vi "要进入系统的界面.vi"() -> ()   [LabVIEW 2015]
panel:
  in  "取消按钮":bool
  in  "声音来源":path=path "E:/桌面/Desktop/wav/儿童歌曲 - 葫芦娃 (儿童版).wav" caption="路径"
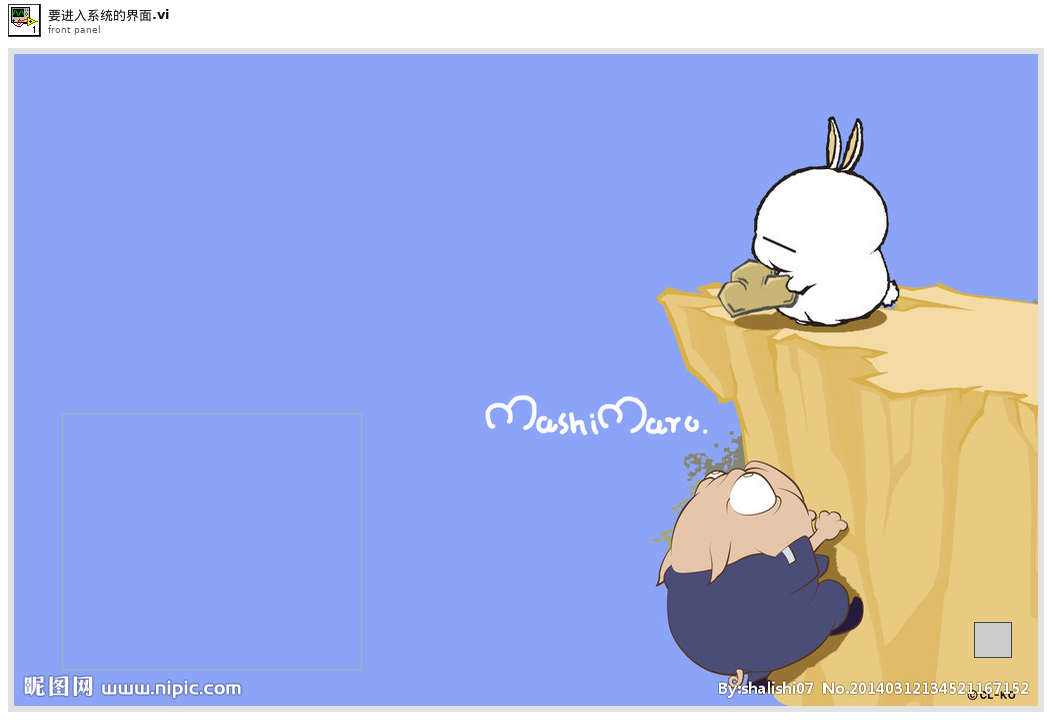
[diagram p1: front panel]
types:
  T1 = typedef "Sound Output Task ID.ctl" = u32
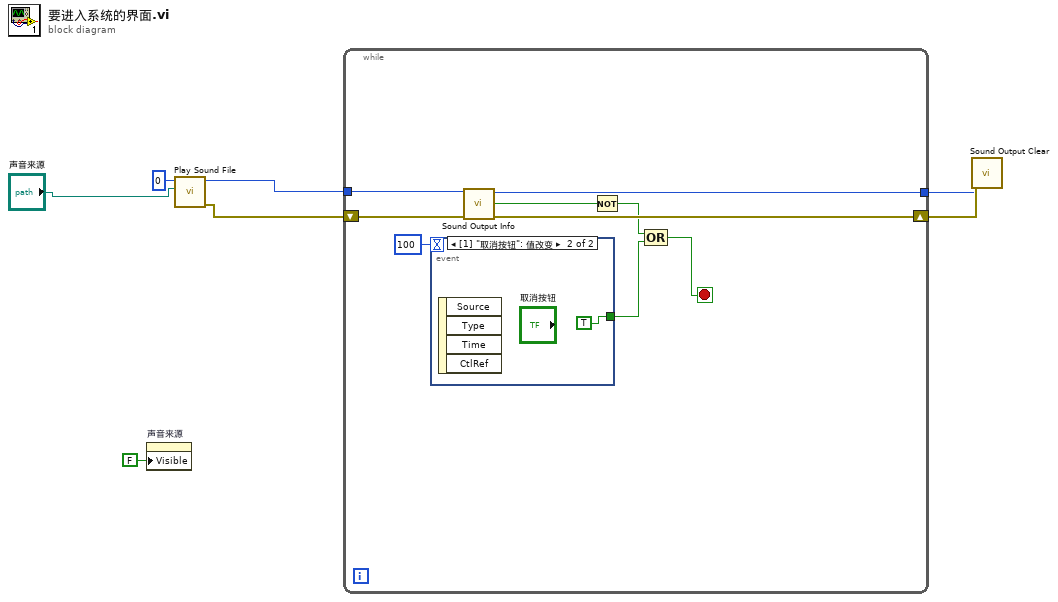
[diagram p0: block diagram]
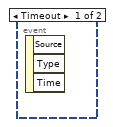
[diagram p2: hidden frame]
diagram:
  n1 = property on="声音来源" class="Path"("Visible"=FALSE ("可见")) -> ()  [unwired: 2 in, 2 out]
  n2 = call <vilib>:"Play Sound File.vi"("path"="声音来源", "device ID"=u32 0) -> ("error out"=w5:errorcluster, "task ID"=w4:T1)  [unwired: 8 in]
  n3 = while {
    tunnel: w4 -> [w16]
    tunnel: [w13] -> w6
    shift-right: [w14] -> w7
    shift-left: w5 -> [w15]
    stop <- w8 stop-if-true
    n4 = event shown="[1] \"取消按钮\": 值改变" {
      selector: _ -> [_ _]
      dyn-events: _ -> [_ _]
      timeout: 100 -> [_ _]
      tunnel: [_ TRUE] -> w9
      event Timeout {
        n5 = event-data() -> ()  [unwired: 1 in, 3 out]
      }
      event "取消按钮": Value Change {
        n6 = event-data() -> ()  [unwired: 1 in, 4 out]
      }
    }
    n7 = call <vilib>:"Sound Output Info.vi"("error in (no error)"=w15, "task ID"=w16) -> ("error out"=w14:errorcluster, "is playing?"=w11:bool, "task ID out"=w13:T1)  [unwired: 6 in, 1 out]
    n8 = Not(x=w11) -> (.not. x?=w12:bool)
    n9 = Compound Arithmetic op=OR(w12, w9) -> (w8:bool)
  }
  n10 = call <vilib>:"Sound Output Clear.vi"("error in (no error)"=w7, "task ID"=w6) -> ()  [unwired: 9 in, 1 out]
